vi "Single IV and Ic distribution.vi"() -> ()   [LabVIEW 2021]
uses:
  RT fast data.ctl
  <vilib>/LabVIEW Targets/FPGA/cRIO/shared/nicrio_ModuleControls/nicrio_cRIO-9775_RecordDataRates4ChansRing.ctl
  <resource>/objmgr/ni.dex.rc
  <vilib>/Analysis/NI_AALBase.lvlib
panel:
  out "output file name":string="20211220-163733-Single IV and DistG16R_Dist.dat"
  out "Threshold":dbl=0.13652587890625
  in  "length":i32=1000
  in  "Begin index":i32=1000
  in  "Tab Control":T1(tab)
  in  "IV Record Samples":u32=5000
  in  "Dist Records Num":i32=10000
  in  "IV Record Data Rate":T2=200 items=["20.000 MS/s (NI 9775)"=1, "10.00 MS/s (NI 9775)"=2, "6.667 MS/s (NI 9775)"=3, "5.000 MS/s (NI 9775)"=4, "2.500 MS/s (NI 9775)"=8, "1.667 MS/s (NI 9775)"=12, "1.250 MS/s (NI 9775)"=16, "1.000 MS/s (NI 9775)"=20, "833.333 KS/s (NI 9775)"=24, "714.286 KS/s (NI 9775)"=28, "625.000 KS/s (NI 9775)"=32, "555.556 KS/s (NI 9775)"=36, "500.000 KS/s (NI 9775)"=40, "454.545 KS/s (NI 9775)"=44, "416.667 KS/s (NI 9775)"=48, "384.615 KS/s (NI 9775)"=52, "357.143 KS/s (NI 9775)"=56, "333.333 KS/s (NI 9775)"=60, "312.500 KS/s (NI 9775)"=64, "294.118 KS/s (NI 9775)"=68, "277.778 KS/s (NI 9775)"=72, "263.158 KS/s (NI 9775)"=76, "250.000 KS/s (NI 9775)"=80, "238.095 KS/s (NI 9775)"=84, "227.273 KS/s (NI 9775)"=88, "217.391 KS/s (NI 9775)"=92, "208.333 KS/s (NI 9775)"=96, "200.000 KS/s (NI 9775)"=100, "192.308 KS/s (NI 9775)"=104, "185.185 KS/s (NI 9775)"=108, "178.571 KS/s (NI 9775)"=112, "172.414 KS/s (NI 9775)"=116, "166.667 KS/s (NI 9775)"=120, "161.290 KS/s (NI 9775)"=124, "156.250 KS/s (NI 9775)"=128, "151.515 KS/s (NI 9775)"=132, "147.059 KS/s (NI 9775)"=136, "142.857 KS/s (NI 9775)"=140, "138.889 KS/s (NI 9775)"=144, "135.135 KS/s (NI 9775)"=148, "131.579 KS/s (NI 9775)"=152, "128.205 KS/s (NI 9775)"=156, "125.000 KS/s (NI 9775)"=160, "121.951 KS/s (NI 9775)"=164, "119.048 KS/s (NI 9775)"=168, "116.279 KS/s (NI 9775)"=172, "113.636 KS/s (NI 9775)"=176, "111.111 KS/s (NI 9775)"=180, "108.696 KS/s (NI 9775)"=184, "106.383 KS/s (NI 9775)"=188, "104.167 KS/s (NI 9775)"=192, "102.041 KS/s (NI 9775)"=196, "100.000 KS/s (NI 9775)"=200, "50.000 KS/s (NI 9775)"=400, "33.333 KS/s (NI 9775)"=600, "25.000 KS/s (NI 9775)"=800, "20.000 KS/s (NI 9775)"=1000, "16.667 KS/s (NI 9775)"=1200, "14.286 KS/s (NI 9775)"=1400, "12.500 KS/s (NI 9775)"=1600, "11.111 KS/s (NI 9775)"=1800, "10.000 KS/s (NI 9775)"=2000, "9.091 KS/s (NI 9775)"=2200, "8.333 KS/s (NI 9775)"=2400, "7.692 KS/s (NI 9775)"=2600, "7.143 KS/s (NI 9775)"=2800, "6.667 KS/s (NI 9775)"=3000, "6.250 KS/s (NI 9775)"=3200, "5.882 KS/s (NI 9775)"=3400, "5.556 KS/s (NI 9775)"=3600, "5.000 KS/s (NI 9775)"=4000, "4.762 KS/s (NI 9775)"=4200, "4.545 KS/s (NI 9775)"=4400, "4.348 KS/s (NI 9775)"=4600, "4.167 KS/s (NI 9775)"=4800, "4.000 KS/s (NI 9775)"=5000, "3.846 KS/s (NI 9775)"=5200, "3.571 KS/s (NI 9775)"=5600, "3.333 KS/s (NI 9775)"=6000, "3.125 KS/s (NI 9775)"=6400, "2.941 KS/s (NI 9775)"=6800, "2.778 KS/s (NI 9775)"=7200, "2.632 KS/s (NI 9775)"=7600, "2.500 KS/s (NI 9775)"=8000, "2.381 KS/s (NI 9775)"=8400, "2.273 KS/s (NI 9775)"=8800, "2.174 KS/s (NI 9775)"=9200, "2.083 KS/s (NI 9775)"=9600, "2.000 KS/s (NI 9775)"=10000, "1.923 KS/s (NI 9775)"=10400, "1.852 KS/s (NI 9775)"=10800, "1.786 KS/s (NI 9775)"=11200, "1.724 KS/s (NI 9775)"=11600, "1.667 KS/s (NI 9775)"=12000, "1.613 KS/s (NI 9775)"=12400, "1.563 KS/s (NI 9775)"=12800, "1.515 KS/s (NI 9775)"=13200, "1.471 KS/s (NI 9775)"=13600, "1.429 KS/s (NI 9775)"=14000, "1.389 KS/s (NI 9775)"=14400, "1.351 KS/s (NI 9775)"=14800, "1.316 KS/s (NI 9775)"=15200, "1.282 KS/s (NI 9775)"=15600, "1.250 KS/s (NI 9775)"=16000, "1.220 KS/s (NI 9775)"=16400, "1.190 KS/s (NI 9775)"=16800, "1.163 KS/s (NI 9775)"=17200, "1.136 KS/s (NI 9775)"=17600, "1.111 KS/s (NI 9775)"=18000, "1.087 KS/s (NI 9775)"=18400, "1.064 KS/s (NI 9775)"=18800, "1.042 KS/s (NI 9775)"=19200, "1.020 KS/s (NI 9775)"=19600, "1.000 KS/s (NI 9775)"=20000, "0.980 KS/s (NI 9775)"=20400, "0.962 KS/s (NI 9775)"=20800, "0.943 KS/s (NI 9775)"=21200, "0.926 KS/s (NI 9775)"=21600, "0.909 KS/s (NI 9775)"=22000, "0.893 KS/s (NI 9775)"=22400, "0.877 KS/s (NI 9775)"=22800, "0.862 KS/s (NI 9775)"=23200, "0.847 KS/s (NI 9775)"=23600, "0.833 KS/s (NI 9775)"=24000, "0.820 KS/s (NI 9775)"=24400, "0.806 KS/s (NI 9775)"=24800, "0.794 KS/s (NI 9775)"=25200, "0.781 KS/s (NI 9775)"=25600, "0.694 KS/s (NI 9775)"=28800, "0.625 KS/s (NI 9775)"=32000, "0.568 KS/s (NI 9775)"=35200, "0.521 KS/s (NI 9775)"=38400, "0.446 KS/s (NI 9775)"=44800, "0.391 KS/s (NI 9775)"=51200, "0.347 KS/s (NI 9775)"=57600, "0.313 KS/s (NI 9775)"=64000]
  in  "Gate wait time us":u32=150
  in  "Current Scale factor":dbl=1.0
  in  "Voltage Scale factor":dbl=0.0001
  in  "Relative Threshold":dbl=0.16
  in  "Read point":i32=1
  in  "Wire resistance":dbl
  in  "Data buffer size":i32=1000
  in  "cRIO IP":string="//172.22.11.2"
  in  "Zero avg":i32=500
  in  "Count us half of T":u32=1
  in  "Wait before trigger us":u32=10100
  in  "Cutoff delay usec":u32=10000
  in  "Tab Control 2":enum32{"IV parameters", "Ic parameters"}(tab)=enum."Ic parameters"
  out "IV parameters":T3={"Records Num"=1, "AI Trigger Configuration"={"Trigger Slope"=enum."Positive", "Trigger Level"=0.10009765625, "Hystesis Value"=0.094970703125, "AI Channel"=0}, "Record PreTrigger Samples"=1, "Record Samples"=5000, "Ic Cut off or curve"=FALSE, "Gate wait time us"=150, "Record Data Rate"=200, "Count us half of T"=1, "Wait before trigger us"=10100, "Cutoff delay usec"=500} {"Record Data Rate" items=["20.000 MS/s (NI 9775)"=1, "10.00 MS/s (NI 9775)"=2, "6.667 MS/s (NI 9775)"=3, "5.000 MS/s (NI 9775)"=4, "2.500 MS/s (NI 9775)"=8, "1.667 MS/s (NI 9775)"=12, "1.250 MS/s (NI 9775)"=16, "1.000 MS/s (NI 9775)"=20, "833.333 KS/s (NI 9775)"=24, "714.286 KS/s (NI 9775)"=28, "625.000 KS/s (NI 9775)"=32, "555.556 KS/s (NI 9775)"=36, "500.000 KS/s (NI 9775)"=40, "454.545 KS/s (NI 9775)"=44, "416.667 KS/s (NI 9775)"=48, "384.615 KS/s (NI 9775)"=52, "357.143 KS/s (NI 9775)"=56, "333.333 KS/s (NI 9775)"=60, "312.500 KS/s (NI 9775)"=64, "294.118 KS/s (NI 9775)"=68, "277.778 KS/s (NI 9775)"=72, "263.158 KS/s (NI 9775)"=76, "250.000 KS/s (NI 9775)"=80, "238.095 KS/s (NI 9775)"=84, "227.273 KS/s (NI 9775)"=88, "217.391 KS/s (NI 9775)"=92, "208.333 KS/s (NI 9775)"=96, "200.000 KS/s (NI 9775)"=100, "192.308 KS/s (NI 9775)"=104, "185.185 KS/s (NI 9775)"=108, "178.571 KS/s (NI 9775)"=112, "172.414 KS/s (NI 9775)"=116, "166.667 KS/s (NI 9775)"=120, "161.290 KS/s (NI 9775)"=124, "156.250 KS/s (NI 9775)"=128, "151.515 KS/s (NI 9775)"=132, "147.059 KS/s (NI 9775)"=136, "142.857 KS/s (NI 9775)"=140, "138.889 KS/s (NI 9775)"=144, "135.135 KS/s (NI 9775)"=148, "131.579 KS/s (NI 9775)"=152, "128.205 KS/s (NI 9775)"=156, "125.000 KS/s (NI 9775)"=160, "121.951 KS/s (NI 9775)"=164, "119.048 KS/s (NI 9775)"=168, "116.279 KS/s (NI 9775)"=172, "113.636 KS/s (NI 9775)"=176, "111.111 KS/s (NI 9775)"=180, "108.696 KS/s (NI 9775)"=184, "106.383 KS/s (NI 9775)"=188, "104.167 KS/s (NI 9775)"=192, "102.041 KS/s (NI 9775)"=196, "100.000 KS/s (NI 9775)"=200, "50.000 KS/s (NI 9775)"=400, "33.333 KS/s (NI 9775)"=600, "25.000 KS/s (NI 9775)"=800, "20.000 KS/s (NI 9775)"=1000, "16.667 KS/s (NI 9775)"=1200, "14.286 KS/s (NI 9775)"=1400, "12.500 KS/s (NI 9775)"=1600, "11.111 KS/s (NI 9775)"=1800, "10.000 KS/s (NI 9775)"=2000, "9.091 KS/s (NI 9775)"=2200, "8.333 KS/s (NI 9775)"=2400, "7.692 KS/s (NI 9775)"=2600, "7.143 KS/s (NI 9775)"=2800, "6.667 KS/s (NI 9775)"=3000, "6.250 KS/s (NI 9775)"=3200, "5.882 KS/s (NI 9775)"=3400, "5.556 KS/s (NI 9775)"=3600, "5.000 KS/s (NI 9775)"=4000, "4.762 KS/s (NI 9775)"=4200, "4.545 KS/s (NI 9775)"=4400, "4.348 KS/s (NI 9775)"=4600, "4.167 KS/s (NI 9775)"=4800, "4.000 KS/s (NI 9775)"=5000, "3.846 KS/s (NI 9775)"=5200, "3.571 KS/s (NI 9775)"=5600, "3.333 KS/s (NI 9775)"=6000, "3.125 KS/s (NI 9775)"=6400, "2.941 KS/s (NI 9775)"=6800, "2.778 KS/s (NI 9775)"=7200, "2.632 KS/s (NI 9775)"=7600, "2.500 KS/s (NI 9775)"=8000, "2.381 KS/s (NI 9775)"=8400, "2.273 KS/s (NI 9775)"=8800, "2.174 KS/s (NI 9775)"=9200, "2.083 KS/s (NI 9775)"=9600, "2.000 KS/s (NI 9775)"=10000, "1.923 KS/s (NI 9775)"=10400, "1.852 KS/s (NI 9775)"=10800, "1.786 KS/s (NI 9775)"=11200, "1.724 KS/s (NI 9775)"=11600, "1.667 KS/s (NI 9775)"=12000, "1.613 KS/s (NI 9775)"=12400, "1.563 KS/s (NI 9775)"=12800, "1.515 KS/s (NI 9775)"=13200, "1.471 KS/s (NI 9775)"=13600, "1.429 KS/s (NI 9775)"=14000, "1.389 KS/s (NI 9775)"=14400, "1.351 KS/s (NI 9775)"=14800, "1.316 KS/s (NI 9775)"=15200, "1.282 KS/s (NI 9775)"=15600, "1.250 KS/s (NI 9775)"=16000, "1.220 KS/s (NI 9775)"=16400, "1.190 KS/s (NI 9775)"=16800, "1.163 KS/s (NI 9775)"=17200, "1.136 KS/s (NI 9775)"=17600, "1.111 KS/s (NI 9775)"=18000, "1.087 KS/s (NI 9775)"=18400, "1.064 KS/s (NI 9775)"=18800, "1.042 KS/s (NI 9775)"=19200, "1.020 KS/s (NI 9775)"=19600, "1.000 KS/s (NI 9775)"=20000, "0.980 KS/s (NI 9775)"=20400, "0.962 KS/s (NI 9775)"=20800, "0.943 KS/s (NI 9775)"=21200, "0.926 KS/s (NI 9775)"=21600, "0.909 KS/s (NI 9775)"=22000, "0.893 KS/s (NI 9775)"=22400, "0.877 KS/s (NI 9775)"=22800, "0.862 KS/s (NI 9775)"=23200, "0.847 KS/s (NI 9775)"=23600, "0.833 KS/s (NI 9775)"=24000, "0.820 KS/s (NI 9775)"=24400, "0.806 KS/s (NI 9775)"=24800, "0.794 KS/s (NI 9775)"=25200, "0.781 KS/s (NI 9775)"=25600, "0.694 KS/s (NI 9775)"=28800, "0.625 KS/s (NI 9775)"=32000, "0.568 KS/s (NI 9775)"=35200, "0.521 KS/s (NI 9775)"=38400, "0.446 KS/s (NI 9775)"=44800, "0.391 KS/s (NI 9775)"=51200, "0.347 KS/s (NI 9775)"=57600, "0.313 KS/s (NI 9775)"=64000]}
  out "Ic parameters":T3={"Records Num"=10000, "AI Trigger Configuration"={"Trigger Slope"=enum."Positive", "Trigger Level"=0.136474609375, "Hystesis Value"=0.0, "AI Channel"=0}, "Record PreTrigger Samples"=1, "Record Samples"=16, "Ic Cut off or curve"=TRUE, "Gate wait time us"=150, "Record Data Rate"=1, "Count us half of T"=1, "Wait before trigger us"=10100, "Cutoff delay usec"=10000} {"Record Data Rate" items=["20.000 MS/s (NI 9775)"=1, "10.00 MS/s (NI 9775)"=2, "6.667 MS/s (NI 9775)"=3, "5.000 MS/s (NI 9775)"=4, "2.500 MS/s (NI 9775)"=8, "1.667 MS/s (NI 9775)"=12, "1.250 MS/s (NI 9775)"=16, "1.000 MS/s (NI 9775)"=20, "833.333 KS/s (NI 9775)"=24, "714.286 KS/s (NI 9775)"=28, "625.000 KS/s (NI 9775)"=32, "555.556 KS/s (NI 9775)"=36, "500.000 KS/s (NI 9775)"=40, "454.545 KS/s (NI 9775)"=44, "416.667 KS/s (NI 9775)"=48, "384.615 KS/s (NI 9775)"=52, "357.143 KS/s (NI 9775)"=56, "333.333 KS/s (NI 9775)"=60, "312.500 KS/s (NI 9775)"=64, "294.118 KS/s (NI 9775)"=68, "277.778 KS/s (NI 9775)"=72, "263.158 KS/s (NI 9775)"=76, "250.000 KS/s (NI 9775)"=80, "238.095 KS/s (NI 9775)"=84, "227.273 KS/s (NI 9775)"=88, "217.391 KS/s (NI 9775)"=92, "208.333 KS/s (NI 9775)"=96, "200.000 KS/s (NI 9775)"=100, "192.308 KS/s (NI 9775)"=104, "185.185 KS/s (NI 9775)"=108, "178.571 KS/s (NI 9775)"=112, "172.414 KS/s (NI 9775)"=116, "166.667 KS/s (NI 9775)"=120, "161.290 KS/s (NI 9775)"=124, "156.250 KS/s (NI 9775)"=128, "151.515 KS/s (NI 9775)"=132, "147.059 KS/s (NI 9775)"=136, "142.857 KS/s (NI 9775)"=140, "138.889 KS/s (NI 9775)"=144, "135.135 KS/s (NI 9775)"=148, "131.579 KS/s (NI 9775)"=152, "128.205 KS/s (NI 9775)"=156, "125.000 KS/s (NI 9775)"=160, "121.951 KS/s (NI 9775)"=164, "119.048 KS/s (NI 9775)"=168, "116.279 KS/s (NI 9775)"=172, "113.636 KS/s (NI 9775)"=176, "111.111 KS/s (NI 9775)"=180, "108.696 KS/s (NI 9775)"=184, "106.383 KS/s (NI 9775)"=188, "104.167 KS/s (NI 9775)"=192, "102.041 KS/s (NI 9775)"=196, "100.000 KS/s (NI 9775)"=200, "50.000 KS/s (NI 9775)"=400, "33.333 KS/s (NI 9775)"=600, "25.000 KS/s (NI 9775)"=800, "20.000 KS/s (NI 9775)"=1000, "16.667 KS/s (NI 9775)"=1200, "14.286 KS/s (NI 9775)"=1400, "12.500 KS/s (NI 9775)"=1600, "11.111 KS/s (NI 9775)"=1800, "10.000 KS/s (NI 9775)"=2000, "9.091 KS/s (NI 9775)"=2200, "8.333 KS/s (NI 9775)"=2400, "7.692 KS/s (NI 9775)"=2600, "7.143 KS/s (NI 9775)"=2800, "6.667 KS/s (NI 9775)"=3000, "6.250 KS/s (NI 9775)"=3200, "5.882 KS/s (NI 9775)"=3400, "5.556 KS/s (NI 9775)"=3600, "5.000 KS/s (NI 9775)"=4000, "4.762 KS/s (NI 9775)"=4200, "4.545 KS/s (NI 9775)"=4400, "4.348 KS/s (NI 9775)"=4600, "4.167 KS/s (NI 9775)"=4800, "4.000 KS/s (NI 9775)"=5000, "3.846 KS/s (NI 9775)"=5200, "3.571 KS/s (NI 9775)"=5600, "3.333 KS/s (NI 9775)"=6000, "3.125 KS/s (NI 9775)"=6400, "2.941 KS/s (NI 9775)"=6800, "2.778 KS/s (NI 9775)"=7200, "2.632 KS/s (NI 9775)"=7600, "2.500 KS/s (NI 9775)"=8000, "2.381 KS/s (NI 9775)"=8400, "2.273 KS/s (NI 9775)"=8800, "2.174 KS/s (NI 9775)"=9200, "2.083 KS/s (NI 9775)"=9600, "2.000 KS/s (NI 9775)"=10000, "1.923 KS/s (NI 9775)"=10400, "1.852 KS/s (NI 9775)"=10800, "1.786 KS/s (NI 9775)"=11200, "1.724 KS/s (NI 9775)"=11600, "1.667 KS/s (NI 9775)"=12000, "1.613 KS/s (NI 9775)"=12400, "1.563 KS/s (NI 9775)"=12800, "1.515 KS/s (NI 9775)"=13200, "1.471 KS/s (NI 9775)"=13600, "1.429 KS/s (NI 9775)"=14000, "1.389 KS/s (NI 9775)"=14400, "1.351 KS/s (NI 9775)"=14800, "1.316 KS/s (NI 9775)"=15200, "1.282 KS/s (NI 9775)"=15600, "1.250 KS/s (NI 9775)"=16000, "1.220 KS/s (NI 9775)"=16400, "1.190 KS/s (NI 9775)"=16800, "1.163 KS/s (NI 9775)"=17200, "1.136 KS/s (NI 9775)"=17600, "1.111 KS/s (NI 9775)"=18000, "1.087 KS/s (NI 9775)"=18400, "1.064 KS/s (NI 9775)"=18800, "1.042 KS/s (NI 9775)"=19200, "1.020 KS/s (NI 9775)"=19600, "1.000 KS/s (NI 9775)"=20000, "0.980 KS/s (NI 9775)"=20400, "0.962 KS/s (NI 9775)"=20800, "0.943 KS/s (NI 9775)"=21200, "0.926 KS/s (NI 9775)"=21600, "0.909 KS/s (NI 9775)"=22000, "0.893 KS/s (NI 9775)"=22400, "0.877 KS/s (NI 9775)"=22800, "0.862 KS/s (NI 9775)"=23200, "0.847 KS/s (NI 9775)"=23600, "0.833 KS/s (NI 9775)"=24000, "0.820 KS/s (NI 9775)"=24400, "0.806 KS/s (NI 9775)"=24800, "0.794 KS/s (NI 9775)"=25200, "0.781 KS/s (NI 9775)"=25600, "0.694 KS/s (NI 9775)"=28800, "0.625 KS/s (NI 9775)"=32000, "0.568 KS/s (NI 9775)"=35200, "0.521 KS/s (NI 9775)"=38400, "0.446 KS/s (NI 9775)"=44800, "0.391 KS/s (NI 9775)"=51200, "0.347 KS/s (NI 9775)"=57600, "0.313 KS/s (NI 9775)"=64000]}
  out "error out":errorcluster
  in  "Sample Name":string="G16R"
  in  "Data folder":path=path "C:/Users/gyue/Desktop/data 20211216"
  out "Time to Init ms":u32=736
  out "Start time ms":u32=342141640
  out "Done":bool=TRUE
  out "Array":dbl[](array[numeric])
  out "Histogram Graph":T4(graph)={"X Values"=[1.591646728515625, 1.5991589355468752, 1.6066711425781253, 1.6141833496093754, 1.6216955566406255, 1.6292077636718756, 1.6367199707031257, 1.6442321777343758, 1.651744384765626, 1.659256591796876, 1.6667687988281261, 1.6742810058593762, 1.6817932128906263, 1.6893054199218764, 1.6968176269531265, 1.7043298339843767, 1.7118420410156268, 1.7193542480468769, 1.726866455078127, 1.734378662109377, 1.7418908691406272, 1.7494030761718773, 1.7569152832031274, 1.7644274902343775, 1.7719396972656276, 1.7794519042968777, 1.7869641113281278, 1.794476318359378, 1.801988525390628, 1.8095007324218781, 1.8170129394531283, 1.8245251464843784, 1.8320373535156285, 1.8395495605468786, 1.8470617675781287, 1.8545739746093788, 1.862086181640629, 1.869598388671879, 1.877110595703129, 1.8846228027343792, 1.8921350097656293, 1.8996472167968794, 1.9071594238281295, 1.9146716308593796, 1.9221838378906297, 1.9296960449218798, 1.93720825195313, 1.94472045898438, 1.9522326660156302, 1.9597448730468803, 1.9672570800781304, 1.9747692871093805, 1.9822814941406306, 1.9897937011718807, 1.9973059082031308, 2.004818115234381, 2.012330322265631, 2.019842529296881, 2.0273547363281312, 2.0348669433593813, 2.0423791503906314, 2.0498913574218816, 2.0574035644531317, 2.0649157714843818, 2.072427978515632, 2.079940185546882, 2.087452392578132, 2.094964599609382, 2.1024768066406323, 2.1099890136718824, 2.1175012207031325, 2.1250134277343826, 2.1325256347656327, 2.140037841796883, 2.147550048828133, 2.155062255859383, 2.162574462890633, 2.1700866699218833, 2.1775988769531334, 2.1851110839843835, 2.1926232910156336, 2.2001354980468837, 2.207647705078134, 2.215159912109384, 2.222672119140634, 2.230184326171884, 2.237696533203134, 2.2452087402343843, 2.2527209472656344, 2.2602331542968845, 2.2677453613281346, 2.2752575683593848, 2.282769775390635, 2.290281982421885, 2.297794189453135, 2.305306396484385, 2.3128186035156353, 2.3203308105468854, 2.3278430175781355, 2.3353552246093856], "Histogram: h(x)"=[1, 0, 0, 0, 0, 0, 0, 0, 0, 0, 0, 0, 0, 0, 0, 0, 0, 0, 0, 0, 0, 0, 0, 0, 0, 0, 0, 0, 0, 0, 0, 0, 0, 0, 0, 0, 0, 0, 0, 0, 1, 3, 3, 3, 9, 9, 9, 11, 17, 14, 24, 27, 26, 51, 66, 78, 56, 104, 171, 129, 194, 200, 271, 262, 371, 346, 368, 474, 417, 557, 412, 518, 535, 364, 555, 443, 460, 327, 337, 343, 229, 274, 207, 187, 91, 137, 71, 44, 68, 46, 30, 14, 12, 7, 9, 5, 1, 1, 0, 1]}
  out "IV Curve":cluster{"Y":dbl[], "Y":dbl[]}[](graph)
  # "Voltage x factor=uA"
  # "Voltage x factor=actual Volt"
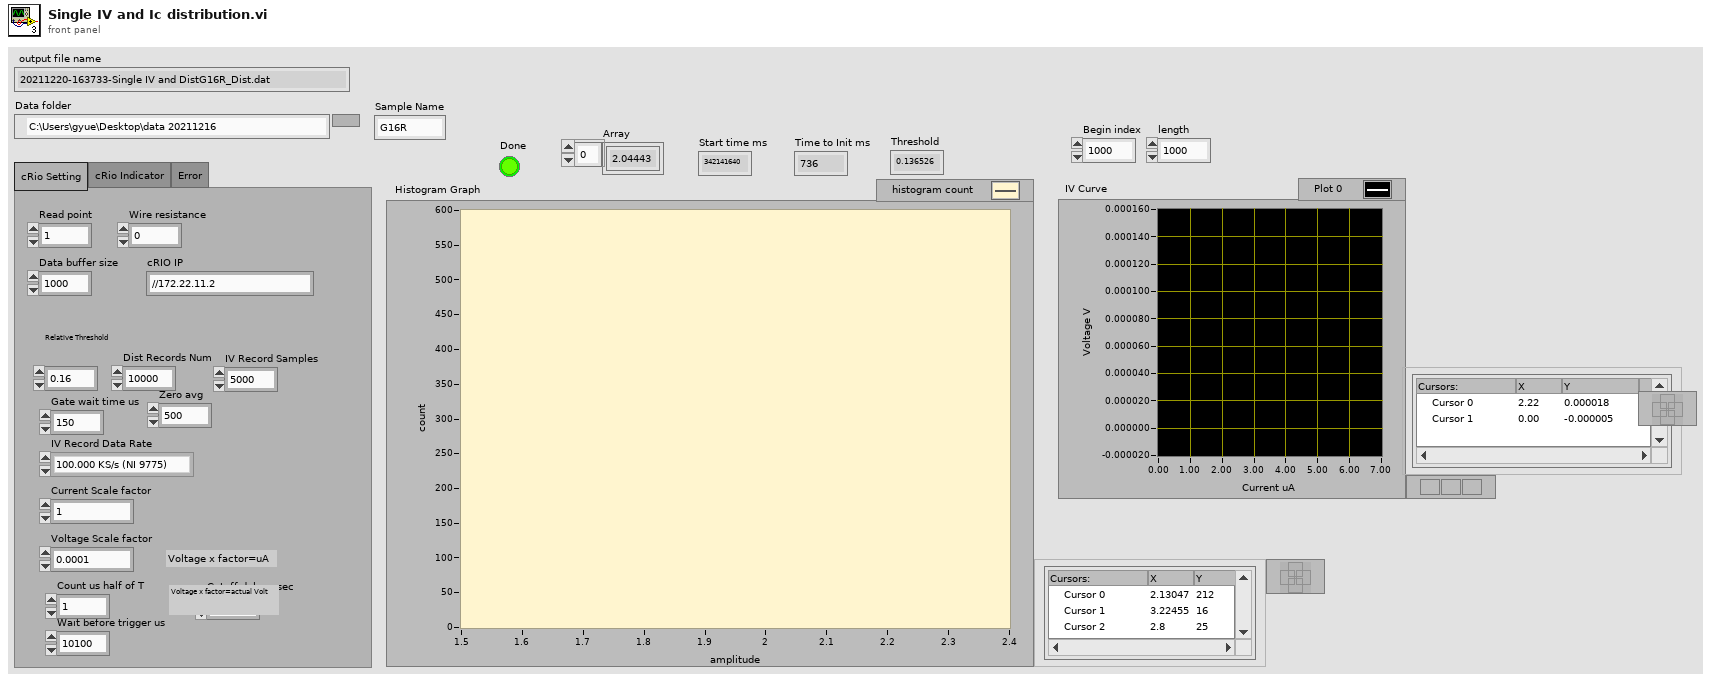
[diagram p1: front panel]
types:
  T1 = enum32{"cRio Setting", "cRio Indicator", "Error"}
  T2 = typedef "nicrio_cRIO-9775_RecordDataRates4ChansRing.ctl" = u16
  T3 = typedef "RT fast data.ctl" = cluster{"Records Num":i32, "AI Trigger Configuration":cluster{"Trigger Slope":enum8{"Positive", "Negative"}, "Trigger Level":fxp<+/-,17,5>, "Hystesis Value":fxp<+,16,4>, "AI Channel":u8}, "Record PreTrigger Samples":u32, "Record Samples":u32, "Ic Cut off or curve":bool, "Gate wait time us":u32, "Record Data Rate":T2, "Count us half of T":u32, "Wait before trigger us":u32, "Cutoff delay usec":u32}
  T4 = cluster{"X Values":dbl[], "Histogram: h(x)":i32[]}
  T5 = cluster{"Trigger Slope":enum8{"Positive", "Negative"}, "Trigger Level":fxp<+/-,17,5>, "Hystesis Value":fxp<+,16,4>, "AI Channel":u8}
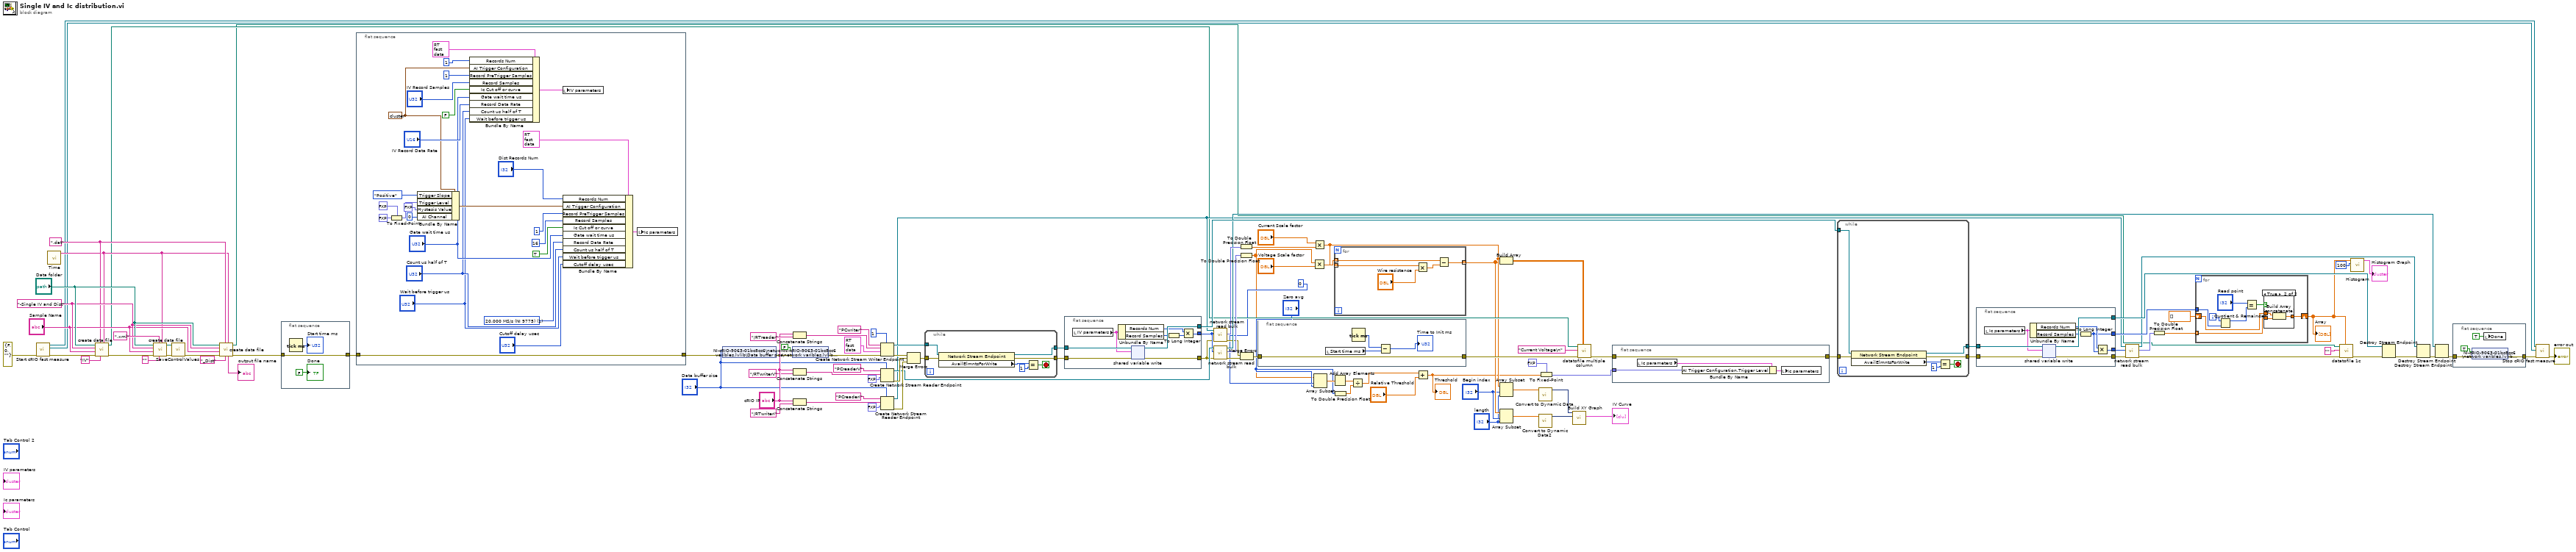
[diagram p0: block diagram]
diagram:
  w47 = ".dat" ("Ext name")
  w49 = "-Single IV and Dist" ("Measurement Name")
  n1 = call "Start cRIO fast measure.vi"("error in (no error)"=errorcluster {"status"=FALSE, "code"=0, "source"=""}) -> ("error out"=w7:errorcluster, "vi reference"=w5:refnum<vi>, "application reference"=w6:refnum<vi>)  [unwired: 8 in]
  n2 = call "Time.vi"() -> ("Timestamp"=w46:string)  [unwired: 11 in]
  n3 = call "create data file.vi"("Time"=w46, "end string"="IV", "Ext name"=w47, "error in (no error)"=w7, "Sample Name"="Sample Name", "Measurement Name"=w49, "base path"="Data folder") -> ("error out"=w55:errorcluster, "appended path"=w45:path)  [unwired: 2 in, 1 out]
  n4 = call "create data file.vi"("Time"=w46, "end string"="", "Ext name"=".xml", "error in (no error)"=w55, "Sample Name"="Sample Name", "Measurement Name"=w49, "base path"="Data folder") -> ("error out"=w34:errorcluster, "appended path"=w35:path)  [unwired: 2 in, 1 out]
  n5 = call "SaveControlValues.vi"("XML File Path"=w35, "error in (no error)"=w34) -> ("error out"=w33:errorcluster)  [unwired: 8 in]
  n6 = call "create data file.vi"("Time"=w46, "end string"="_Dist", "Ext name"=w47, "error in (no error)"=w33, "Sample Name"="Sample Name", "Measurement Name"=w49, "base path"="Data folder") -> ("error out"=w52:errorcluster, "appended path"=w41:path, "file name"=→"output file name":string)  [unwired: 2 in]
  n7 = flat-sequence {
    tunnel: [w111] -> w32
    tunnel: w52 -> [w111]
    frame #0 {
      n8 = Tick Count (ms)() -> (millisecond timer value=→"Start time ms":u32)
      "Done" <- FALSE ("Done")
    }
  }
  n9 = flat-sequence {
    tunnel: w32 -> [w132]
    tunnel: [w132] -> w31
    frame #0 {
      w117 = T2 1 items=["20.000 MS/s (NI 9775)"=1, "10.00 MS/s (NI 9775)"=2, "6.667 MS/s (NI 9775)"=3, "5.000 MS/s (NI 9775)"=4, "2.500 MS/s (NI 9775)"=8, "1.667 MS/s (NI 9775)"=12, "1.250 MS/s (NI 9775)"=16, "1.000 MS/s (NI 9775)"=20, "833.333 KS/s (NI 9775)"=24, "714.286 KS/s (NI 9775)"=28, "625.000 KS/s (NI 9775)"=32, "555.556 KS/s (NI 9775)"=36, "500.000 KS/s (NI 9775)"=40, "454.545 KS/s (NI 9775)"=44, "416.667 KS/s (NI 9775)"=48, "384.615 KS/s (NI 9775)"=52, "357.143 KS/s (NI 9775)"=56, "333.333 KS/s (NI 9775)"=60, "312.500 KS/s (NI 9775)"=64, "294.118 KS/s (NI 9775)"=68, "277.778 KS/s (NI 9775)"=72, "263.158 KS/s (NI 9775)"=76, "250.000 KS/s (NI 9775)"=80, "238.095 KS/s (NI 9775)"=84, "227.273 KS/s (NI 9775)"=88, "217.391 KS/s (NI 9775)"=92, "208.333 KS/s (NI 9775)"=96, "200.000 KS/s (NI 9775)"=100, "192.308 KS/s (NI 9775)"=104, "185.185 KS/s (NI 9775)"=108, "178.571 KS/s (NI 9775)"=112, "172.414 KS/s (NI 9775)"=116, "166.667 KS/s (NI 9775)"=120, "161.290 KS/s (NI 9775)"=124, "156.250 KS/s (NI 9775)"=128, "151.515 KS/s (NI 9775)"=132, "147.059 KS/s (NI 9775)"=136, "142.857 KS/s (NI 9775)"=140, "138.889 KS/s (NI 9775)"=144, "135.135 KS/s (NI 9775)"=148, "131.579 KS/s (NI 9775)"=152, "128.205 KS/s (NI 9775)"=156, "125.000 KS/s (NI 9775)"=160, "121.951 KS/s (NI 9775)"=164, "119.048 KS/s (NI 9775)"=168, "116.279 KS/s (NI 9775)"=172, "113.636 KS/s (NI 9775)"=176, "111.111 KS/s (NI 9775)"=180, "108.696 KS/s (NI 9775)"=184, "106.383 KS/s (NI 9775)"=188, "104.167 KS/s (NI 9775)"=192, "102.041 KS/s (NI 9775)"=196, "100.000 KS/s (NI 9775)"=200, "50.000 KS/s (NI 9775)"=400, "33.333 KS/s (NI 9775)"=600, "25.000 KS/s (NI 9775)"=800, "20.000 KS/s (NI 9775)"=1000, "16.667 KS/s (NI 9775)"=1200, "14.286 KS/s (NI 9775)"=1400, "12.500 KS/s (NI 9775)"=1600, "11.111 KS/s (NI 9775)"=1800, "10.000 KS/s (NI 9775)"=2000, "9.091 KS/s (NI 9775)"=2200, "8.333 KS/s (NI 9775)"=2400, "7.692 KS/s (NI 9775)"=2600, "7.143 KS/s (NI 9775)"=2800, "6.667 KS/s (NI 9775)"=3000, "6.250 KS/s (NI 9775)"=3200, "5.882 KS/s (NI 9775)"=3400, "5.556 KS/s (NI 9775)"=3600, "5.000 KS/s (NI 9775)"=4000, "4.762 KS/s (NI 9775)"=4200, "4.545 KS/s (NI 9775)"=4400, "4.348 KS/s (NI 9775)"=4600, "4.167 KS/s (NI 9775)"=4800, "4.000 KS/s (NI 9775)"=5000, "3.846 KS/s (NI 9775)"=5200, "3.571 KS/s (NI 9775)"=5600, "3.333 KS/s (NI 9775)"=6000, "3.125 KS/s (NI 9775)"=6400, "2.941 KS/s (NI 9775)"=6800, "2.778 KS/s (NI 9775)"=7200, "2.632 KS/s (NI 9775)"=7600, "2.500 KS/s (NI 9775)"=8000, "2.381 KS/s (NI 9775)"=8400, "2.273 KS/s (NI 9775)"=8800, "2.174 KS/s (NI 9775)"=9200, "2.083 KS/s (NI 9775)"=9600, "2.000 KS/s (NI 9775)"=10000, "1.923 KS/s (NI 9775)"=10400, "1.852 KS/s (NI 9775)"=10800, "1.786 KS/s (NI 9775)"=11200, "1.724 KS/s (NI 9775)"=11600, "1.667 KS/s (NI 9775)"=12000, "1.613 KS/s (NI 9775)"=12400, "1.563 KS/s (NI 9775)"=12800, "1.515 KS/s (NI 9775)"=13200, "1.471 KS/s (NI 9775)"=13600, "1.429 KS/s (NI 9775)"=14000, "1.389 KS/s (NI 9775)"=14400, "1.351 KS/s (NI 9775)"=14800, "1.316 KS/s (NI 9775)"=15200, "1.282 KS/s (NI 9775)"=15600, "1.250 KS/s (NI 9775)"=16000, "1.220 KS/s (NI 9775)"=16400, "1.190 KS/s (NI 9775)"=16800, "1.163 KS/s (NI 9775)"=17200, "1.136 KS/s (NI 9775)"=17600, "1.111 KS/s (NI 9775)"=18000, "1.087 KS/s (NI 9775)"=18400, "1.064 KS/s (NI 9775)"=18800, "1.042 KS/s (NI 9775)"=19200, "1.020 KS/s (NI 9775)"=19600, "1.000 KS/s (NI 9775)"=20000, "0.980 KS/s (NI 9775)"=20400, "0.962 KS/s (NI 9775)"=20800, "0.943 KS/s (NI 9775)"=21200, "0.926 KS/s (NI 9775)"=21600, "0.909 KS/s (NI 9775)"=22000, "0.893 KS/s (NI 9775)"=22400, "0.877 KS/s (NI 9775)"=22800, "0.862 KS/s (NI 9775)"=23200, "0.847 KS/s (NI 9775)"=23600, "0.833 KS/s (NI 9775)"=24000, "0.820 KS/s (NI 9775)"=24400, "0.806 KS/s (NI 9775)"=24800, "0.794 KS/s (NI 9775)"=25200, "0.781 KS/s (NI 9775)"=25600, "0.694 KS/s (NI 9775)"=28800, "0.625 KS/s (NI 9775)"=32000, "0.568 KS/s (NI 9775)"=35200, "0.521 KS/s (NI 9775)"=38400, "0.446 KS/s (NI 9775)"=44800, "0.391 KS/s (NI 9775)"=51200, "0.347 KS/s (NI 9775)"=57600, "0.313 KS/s (NI 9775)"=64000] ("Record Data Rate")
      w126 = T5 {"Trigger Slope"=enum."Positive", "Trigger Level"=0.10009765625, "Hystesis Value"=0.094970703125, "AI Channel"=0} ("AI Trigger Configuration")
      n10 = To Fixed-Point(fixed-point type=fxp<+/-,17,5> 0.0 ("Trigger Level"), number=fxp<+/-,32,16> 0.0) -> (fixed-point=w123:fxp<+/-,17,5>)
      n11 = Bundle By Name(cluster=w126, "Trigger Slope"=enum8{"Positive", "Negative"}."Positive", "Trigger Level"=w123, "Hystesis Value"=fxp<+,16,4> 0.0, "AI Channel"=u8 0) -> (w120:T5)
      n12 = Bundle By Name(cluster=T3 {"Records Num"=1, "AI Trigger Configuration"={"Trigger Slope"=enum."Positive", "Trigger Level"=0.10009765625, "Hystesis Value"=0.094970703125, "AI Channel"=0}, "Record PreTrigger Samples"=1, "Record Samples"=5000, "Ic Cut off or curve"=FALSE, "Gate wait time us"=150, "Record Data Rate"=200, "Count us half of T"=15, "Wait before trigger us"=10100, "Cutoff delay usec"=500} ("IV parameters 2"), "Records Num"=1, "AI Trigger Configuration"=w126, "Record PreTrigger Samples"=u32 1, "Record Samples"="IV Record Samples", "Ic Cut off or curve"=FALSE, "Gate wait time us"="Gate wait time us", "Record Data Rate"="IV Record Data Rate", "Count us half of T"="Count us half of T", "Wait before trigger us"="Wait before trigger us") -> (w139:T3)
      n13 = local write "IV parameters"(w139) -> ()
      n14 = Bundle By Name(cluster=T3 {"Records Num"=1, "AI Trigger Configuration"={"Trigger Slope"=enum."Positive", "Trigger Level"=0.10009765625, "Hystesis Value"=0.094970703125, "AI Channel"=0}, "Record PreTrigger Samples"=1, "Record Samples"=5000, "Ic Cut off or curve"=FALSE, "Gate wait time us"=150, "Record Data Rate"=200, "Count us half of T"=15, "Wait before trigger us"=10100, "Cutoff delay usec"=500} ("IV parameters 2"), "Records Num"="Dist Records Num", "AI Trigger Configuration"=w120, "Record PreTrigger Samples"=u32 1, "Record Samples"=u32 16, "Ic Cut off or curve"=TRUE, "Gate wait time us"="Gate wait time us", "Record Data Rate"=w117, "Count us half of T"="Count us half of T", "Wait before trigger us"="Wait before trigger us", "Cutoff delay usec"="Cutoff delay usec") -> (w131:T3)
      n15 = local write "Ic parameters"(w131) -> ()
    }
  }
  n16 = shared-variable "NI-cRIO-9063-01bc8cc6\\network varibles.lvlib\\Data buffer size"("Data buffer size", error in=w31) -> (error out=w87:errorcluster)
  n17 = shared-variable "NI-cRIO-9063-01bc8cc6\\network varibles.lvlib\\RT Stop"(FALSE ("RT Stop"), error in=w87) -> (error out=w94:errorcluster)
  n18 = Concatenate Strings("cRIO IP", "/RTreader" ("string")) -> (w104:string)
  n19 = Concatenate Strings("cRIO IP", "/RTwriterV" ("string")) -> (w96:string)
  n20 = Concatenate Strings("cRIO IP", "/RTwriterI" ("string")) -> (w89:string)
  n21 = Create Network Stream Writer Endpoint(7:1 ("writer buffer size"), 8:w94, 9:T3 {"Records Num"=0, "AI Trigger Configuration"={"Trigger Slope"=enum."Positive", "Trigger Level"=0.0, "Hystesis Value"=0.0, "AI Channel"=0}, "Record PreTrigger Samples"=0, "Record Samples"=0, "Ic Cut off or curve"=FALSE, "Gate wait time us"=0, "Record Data Rate"=1, "Count us half of T"=15, "Wait before trigger us"=10100, "Cutoff delay usec"=500} ("Parameters 4"), 10:w104, 11:"PCwriter" ("writer name")) -> (0:w102:errorcluster, 3:w101:refnum<k21>)  [unwired: 2 in]
  n22 = Create Network Stream Reader Endpoint(7:"Data buffer size", 9:fxp<+/-,17,5> 0.0, 10:w96, 11:"PCreaderV" ("reader name")) -> (0:w93:errorcluster, 3:w66:refnum<k21>)  [unwired: 3 in]
  n23 = Create Network Stream Reader Endpoint(7:"Data buffer size", 9:fxp<+/-,17,5> 0.0, 10:w89, 11:"PCreaderI" ("reader name")) -> (0:w86:errorcluster, 3:w61:refnum<k21>)  [unwired: 3 in]
  n24 = Merge Errors(w102, w93, w86) -> (w100:errorcluster)
  n25 = while {
    tunnel: w101 -> [w146]
    tunnel: w100 -> [w145]
    tunnel: [w141] -> w106
    tunnel: [w140] -> w70
    stop <- w142 stop-if-true
    n26 = property class="Network Stream Endpoint"(reference=w146, error in=w145) -> (reference out=w141:refnum<k21>, error out=w140:errorcluster, "AvailElmntsForWrite"=w144:i32)
    n27 = Equal?(x=w144, y=1) -> (x = y?=w142:bool)
  }
  n28 = flat-sequence {
    tunnel: w106 -> [w155]
    tunnel: [w154] -> w83
    tunnel: w70 -> [w150]
    tunnel: [w149] -> w65
    tunnel: [w148] -> w56
    frame #0 {
      n29 = local read "IV parameters"() -> (w147:T3)
      n30 = Unbundle By Name(w147) -> ("Records Num"=w153:i32, "Record Samples"=w152:u32)
      n31 = shared-variable-write(w155, w150, w147) -> (w154:refnum<k21>, w148:errorcluster)  [unwired: 1 in, 1 out]
      n32 = To Long Integer(number=w152) -> (32bit integer=w151:i32)
      n33 = Multiply(x=w153, y=w151) -> (x*y=w149:i32)
    }
  }
  n34 = call "network stream read bulk.vi"("endpoint in"=w61, "Data num"=w65, "error in (no error)"=w56) -> ("Data"=w68:fxp<+/-,17,5>[], "error out"=w63:errorcluster)  [unwired: 5 in, 1 out]
  n35 = call "network stream read bulk.vi"("endpoint in"=w66, "Data num"=w65, "error in (no error)"=w56) -> ("endpoint out"=w64:refnum<k21>, "Data"=w67:fxp<+/-,17,5>[], "error out"=w62:errorcluster)  [unwired: 5 in]
  n36 = To Double Precision Float(number=w68) -> (double precision float=w29:dbl[])
  n37 = To Double Precision Float(number=w67) -> (double precision float=w12:dbl[])
  n38 = Merge Errors(w63, w62) -> (w69:errorcluster)
  n39 = flat-sequence {
    tunnel: w69 -> [w156]
    tunnel: [w156] -> w42
    frame #0 {
      n40 = local read "Start time ms"() -> (w158:u32)
      n41 = Tick Count (ms)() -> (millisecond timer value=w159:u32)
      n42 = Subtract(x=w159, y=w158) -> (x-y=→"Time to Init ms":u32)
    }
  }
  n43 = Multiply(x=w12, y="Voltage Scale factor") -> (x*y=w27:dbl[])
  n44 = Multiply(x="Current Scale factor", y=w29) -> (x*y=w26:dbl[])
  n45 = Array Subset(array=w12, index=0, length="Zero avg") -> (w19:dbl[])
  n46 = Add Array Elements(numeric array=w19) -> (sum=w18:dbl)
  n47 = To Double Precision Float(number="Zero avg") -> (double precision float=w16:dbl)
  n48 = for {
    tunnel: w27 -> [w164] mode=indexing
    tunnel: w26 -> [w162] mode=indexing
    tunnel: [w160] -> w24 mode=indexing
    n49 = Multiply(x=w162, y="Wire resistance") -> (x*y=w161:dbl)
    n50 = Subtract(x=w164, y=w161) -> (x-y=w160:dbl)
  }
  n51 = Divide(x=w18, y=w16) -> (x/y=w15:dbl)
  n52 = Add(x=w15, y="Relative Threshold") -> (x+y=w13:dbl)
  "Threshold" <- w13
  n53 = Build Array(w26, w24) -> (w43:dbl[][])
  n54 = Array Subset(array=w26, index="Begin index", length="length") -> (w25:dbl[])
  n55 = Array Subset(array=w24, index="Begin index", length="length") -> (w23:dbl[])
  n56 = call "Convert to Dynamic Data"("Array"=w25) -> ("Dynamic Data Type"=w78:dynamicdata)  [unwired: 3 in]
  n57 = call "Convert to Dynamic Data2"("Array"=w23) -> ("Dynamic Data Type"=w77:dynamicdata)  [unwired: 3 in]
  n58 = To Fixed-Point(fixed-point type=fxp<+,16,4> 0.0 ("AI Trigger Configuration.Hystesis Value"), number=w13) -> (fixed-point=w1:fxp<+,16,4>)
  n59 = call "Build XY Graph"("Y Input"=w77, "X Input"=w78) -> ("XY Graph"=→"IV Curve":cluster{"X":dbl[], "Y":dbl[]}[])  [unwired: 8 in, 1 out]
  n60 = call "datatofile multiple column.vi"("2D data"=w43, "error in"=w42, "title"="Current Voltage\n", "file path (dialog if empty)"=w45) -> ("error out"=w10:errorcluster)  [unwired: 7 in]
  n61 = flat-sequence {
    tunnel: w10 -> [w168]
    tunnel: [w168] -> w9
    tunnel: w1 -> [w167]
    frame #0 {
      n62 = local read "Ic parameters"() -> (w165:T3)
      n63 = Bundle By Name(cluster=w165, "AI Trigger Configuration.Trigger Level"=w167) -> (w166:T3)
      n64 = local write "Ic parameters"(w166) -> ()
    }
  }
  n65 = while {
    tunnel: w83 -> [w173]
    tunnel: w9 -> [w172]
    tunnel: [w170] -> w82
    tunnel: [w169] -> w81
    stop <- w171 stop-if-true
    n66 = property class="Network Stream Endpoint"(reference=w173, error in=w172) -> (reference out=w170:refnum<k21>, error out=w169:errorcluster, "AvailElmntsForWrite"=w175:i32)
    n67 = Equal?(x=w175, y=1) -> (x = y?=w171:bool)
  }
  n68 = flat-sequence {
    tunnel: w82 -> [w184]
    tunnel: w81 -> [w183]
    tunnel: [w182] -> w79
    tunnel: [w178] -> w72
    tunnel: [w177] -> w58
    tunnel: [w176] -> w57
    frame #0 {
      n69 = local read "Ic parameters"() -> (w181:T3)
      n70 = Unbundle By Name(w181) -> ("Records Num"=w180:i32, "Record Samples"=w179:u32)
      n71 = shared-variable-write(w184, w183, w181) -> (w182:refnum<k21>, w177:errorcluster)  [unwired: 1 in, 1 out]
      n72 = To Long Integer(number=w179) -> (32bit integer=w178:i32)
      n73 = Multiply(x=w180, y=w178) -> (x*y=w176:i32)
    }
  }
  n74 = call "network stream read bulk.vi"("endpoint in"=w61, "Data num"=w57, "error in (no error)"=w58) -> ("endpoint out"=w60:refnum<k21>, "Data"=w59:fxp<+/-,17,5>[], "error out"=w38:errorcluster)  [unwired: 5 in]
  n75 = To Double Precision Float(number=w59) -> (double precision float=w73:dbl[])
  n76 = for {
    tunnel: w73 -> [w186] mode=indexing
    tunnel: w72 -> [w192]
    shift-right: [w188] -> w36
    shift-left: dbl[] [] -> [w187]
    i -> [w191]
    n77 = Quotient & Remainder(x=w191, y=w192) -> (x-y*floor(x/y)=w190:i32)  [unwired: 1 out]
    n78 = Equal?(x="Read point", y=w190) -> (x = y?=w185:bool)
    n79 = case shown="True" w185 {
      tunnel: [w193 w196] -> w188
      tunnel: w187 -> [w193 w195]
      tunnel: w186 -> [_ w194]
      frame False {
      }
      frame True {
        n80 = Build Array (concatenate)(w195, w194) -> (w196:dbl[])
      }
    }
  }
  "Array" <- w36
  n81 = call "datatofile 1c.vi"("A1"=w36, "error in"=w38, "title"="", "file path (dialog if empty)"=w41) -> ("error out"=w37:errorcluster)  [unwired: 7 in]
  n82 = call <vilib>:"Histogram.vi"("intervals"=100, "X"=w36) -> ("Histogram Graph"=→"Histogram Graph":T4)  [unwired: 6 in, 3 out]
  n83 = Destroy Stream Endpoint(8:w37, 11:w79) -> (0:w92:errorcluster)
  n84 = Destroy Stream Endpoint(8:w92, 11:w60) -> (0:w85:errorcluster)
  n85 = Destroy Stream Endpoint(8:w85, 11:w64) -> (0:w84:errorcluster)
  n86 = flat-sequence {
    tunnel: [w200] -> w4
    tunnel: w84 -> [w199]
    frame #0 {
      n87 = shared-variable "NI-cRIO-9063-01bc8cc6\\network varibles.lvlib\\RT Stop"(TRUE ("RT Stop"), error in=w199) -> (error out=w200:errorcluster)
      n88 = local write "Done"(TRUE ("Done")) -> ()
    }
  }
  n89 = call "Stop cRIO fast measure.vi"("error in (no error)"=w4, "VI reference"=w5, "application reference"=w6) -> ("error out"=→"error out":errorcluster)  [unwired: 8 in]
